vi "MoveScroll.vi"(10 "Text":string, 11 "VI输入":refnum<vi>) -> ()   [LabVIEW 2018]
doc: "将vi的垂直滚动条位置移动到所给定的文本装置控件坐标处"
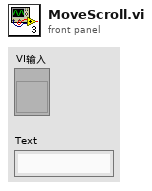
[diagram p1: front panel]
types:
  T1 = typedef "LVPointTypeDef.ctl" = cluster{"Horizontal":i16, "Vertical":i16}
  T2 = typedef "LVPositionTypeDef.ctl" = cluster{"Left":i32, "Top":i32}
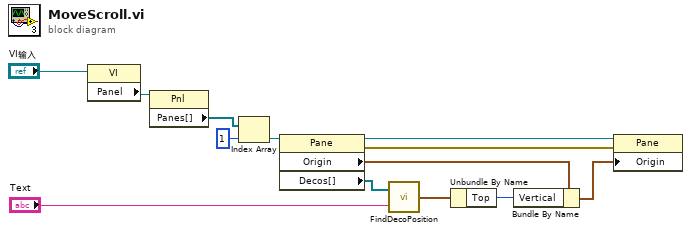
[diagram p0: block diagram]
diagram:
  n1 = property class="VI"(reference="VI输入") -> ("Panel"=w1:refnum<vi>)  [unwired: 1 in, 2 out]
  n2 = property class="Pnl"(reference=w1) -> ("Panes[]"=w2:refnum<vi>[])  [unwired: 1 in, 2 out]
  n3 = Index Array(array=w2, index=1 ("索引")) -> (element=w3:refnum<vi>)
  n4 = property class="Pane"(reference=w3) -> (reference out=w8:refnum<vi>, error out=w7:errorcluster, "Origin"=w5:T1, "Decos[]"=w9:refnum<vi>[])  [unwired: 1 in]
  n5 = call "FindDecoPosition.vi"("Text"="Text", "Decos[]"=w9) -> ("Position"=w11:T2)
  n6 = Unbundle By Name(w11) -> ("Top"=w12:i32)
  n7 = Bundle By Name(cluster=w5, "Vertical"=w12) -> (w6:T1)
  n8 = property class="Pane"(reference=w8, error in=w7, "Origin"=w6) -> ()  [unwired: 2 out]
